vi "RSNRPZ Set Statistics Scale Points.vi"(8 "error in (no error)":errorcluster, 9 "Points (200)":i32=200, 10 "Channel (1)":i32=1, 11 "VISA session":refnum<visa-resource-name> caption="VISA resource name") -> (0 "error out":errorcluster, 3 "dup VISA session":refnum<visa-resource-name> caption="VISA resource name")   [LabVIEW 2010]
doc: "This VI sets the measurement-result resolution in both Statistics modes. This VI specifies the number of pixels that are to be assigned to the logarithmic level range (rsnrpz_stat_setScaleRange VI) for measured value output. The width of the level range divided by N-1, where N is the number of pixels, must not be less than the value which can be read out with rsnrpz_stat_getScaleWidth.\n\nRemote-control command(s):\nSENSe:STATistics:SCALE:X:POINts"
uses:
  rsnrpz_32.dll
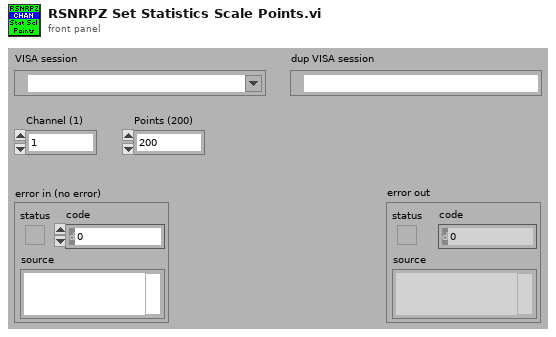
[diagram p1: front panel]
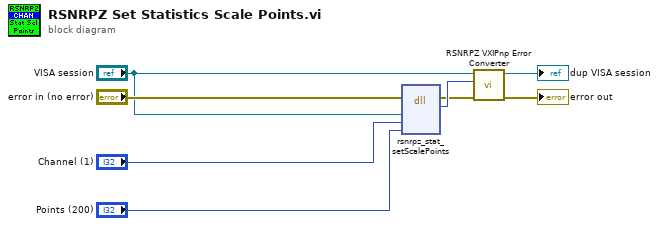
[diagram p0: block diagram]
diagram:
  n1 = dll-call lib="rsnrpz_32.dll" fn="rsnrpz_stat_setScalePoints"(error in="error in (no error)", "Instrument Handle"="VISA session", "Channel"="Channel (1)", "Points"="Points (200)") -> (error out=w5:errorcluster, "Status"=w8:i32)  [unwired: 5 in, 1 out]
  n2 = call <instrlib>:"RSNRPZ VXIPnp Error Converter.vi"("error in"=w5, "VXIPnp error code"=w8, "VISA session"="VISA session") -> ("error out"=→"error out":errorcluster, "dup VISA session"=→"dup VISA session":refnum<visa-resource-name>)  [unwired: 7 in]
